vi "Get idle interval.vi"(8 "error in (no error)":errorcluster, 11 "niDTS WLAN Dut in":refnum<class "niDTS WLAN Dut.lvclass">) -> (0 "error out":errorcluster, 2 "idle interval":dbl=0.0002 format="%_3p", 3 "niDTS WLAN Dut out":refnum<class "niDTS WLAN Dut.lvclass">)   [LabVIEW 2015, in "niDTS WLAN.lvlib" / "niDTS WLAN Dut.lvclass"]
doc: "Gets the Idle Inverval in seconds (s)."
uses:
  niDTS WLAN Dut.lvclass
  niDTS WLAN Dut.lvclass/niDTS WLAN Dut.ctl
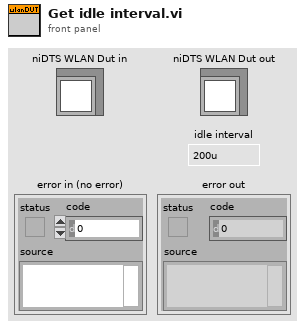
[diagram p1: front panel]
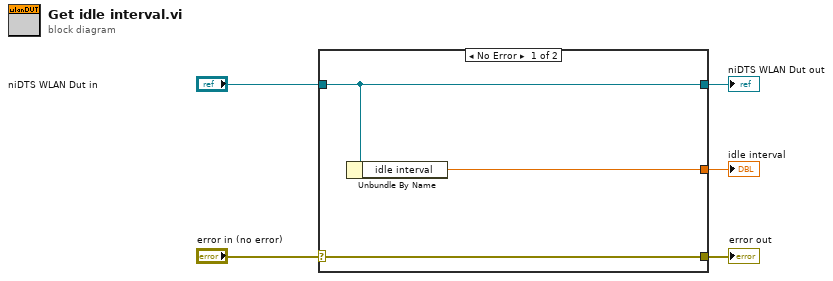
[diagram p0: block diagram]
diagram:
  n1 = case shown="No Error" "error in (no error)" {
    selector: "error in (no error)" -> [w8 w9]
    tunnel: [w8 w9] -> w4
    tunnel: [w7 w10] -> w2
    tunnel: "niDTS WLAN Dut in" -> [w7 w10]
    tunnel: [w6 _] -> w1
    frame No Error {
      n2 = Unbundle By Name(w7) -> ("idle interval"=w6:dbl)
    }
    frame Error {
    }
  }
  "error out" <- w4
  "niDTS WLAN Dut out" <- w2
  "idle interval" <- w1
